vi "write_FP_data_to_fpga.vi"(8 "error in":errorcluster, 10 "all rows":dbl[](array[numeric]), 11 "FPGA Interface":T1) -> (0 "error out":errorcluster, 3 "elements left":i32=1)   [LabVIEW 2017]
uses:
  fpga_interface_types/HOST_to_FPGA_fp_FIFO_interface.ctl
  <vilib>/Utility/error.llb/Error Cluster From Error Code.vi
  <vilib>/rvi/errors/niLvFpgaAdjustHostInterfaceError.vi
  <vilib>/rvi/interface/nirviMethod/nirviMethod.xnode
  <vilib>/FPGAPlugInAG/Dynamic/niLvFpga_WriteFifo_Dynamic.vi
  <vilib>/rvi/errors/niLvFpgaMergeErrorWithErrorCode.vi
panel:
  out "Numeric":i32
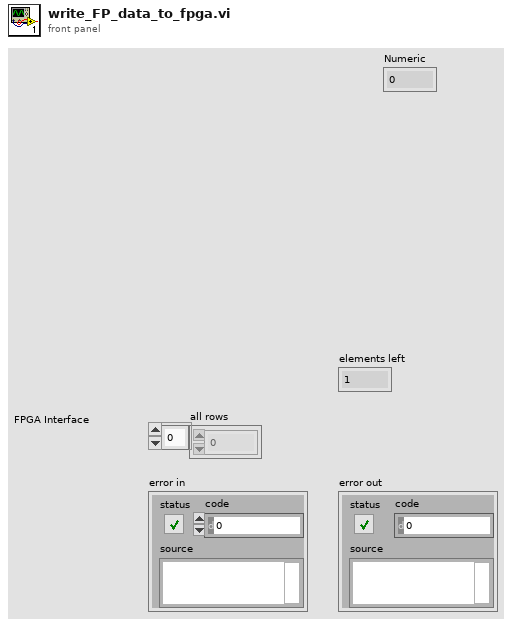
[diagram p1: front panel]
types:
  T1 = typedef "HOST_to_FPGA_fp_FIFO_interface.ctl" = refnum<k20>
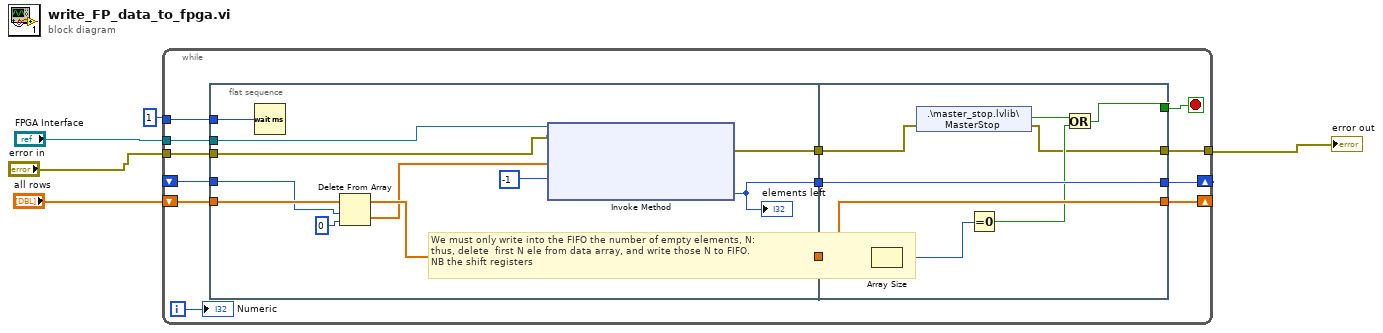
[diagram p0: block diagram]
diagram:
  n1 = while {
    tunnel: [w16] -> w4
    tunnel: 1 -> [w18]
    shift-right: [w11] -> _
    shift-left: _ -> [w15]
    shift-right: [w9] -> _
    shift-left: "all rows" -> [w17]
    tunnel: "FPGA Interface" -> [w8]
    tunnel: "error in" -> [w7]
    i -> [w6]
    stop <- w12 stop-if-true
    n2 = flat-sequence {
      tunnel: w18 -> [w29]
      tunnel: w17 -> [w26]
      tunnel: w15 -> [w25]
      tunnel: [w23] -> w14
      tunnel: [w20] -> w13
      tunnel: [w27] -> w10
      tunnel: w8 -> [w24]
      tunnel: w7 -> [w22]
      tunnel: [w37] -> w11
      tunnel: [w30] -> w16
      tunnel: w14 -> [w31]
      tunnel: w13 -> [w37]
      tunnel: [w33] -> w12
      tunnel: w10 -> [w35]
      tunnel: [w35] -> w9
      frame #0 {
        # "We must only write into the FIFO the number of empty elements, N:\nthus, delete  first N ele from data array, and write those N to FIFO.\nNB the shift registers"
        n3 = Wait (ms)(milliseconds to wait=w29) -> ()  [unwired: 1 out]
        n4 = Delete From Array(array=w26, length=w25, index=0) -> (deleted portion=w19:dbl[], array with subset deleted=w27:dbl[])
        n5 = xnode "Invoke Method"("FPGA VI Reference In"=w24, "error in"=w22, "Data"=w19, "Timeout (ms)"=-1) -> ("error out"=w23:errorcluster, "Empty Elements Remaining"=w20:u32)  [unwired: 1 out]
        "elements left" <- w20
      }
      frame #1 {
        n6 = Array Size(array=w35) -> (size(s)=w36:i32)
        n7 = shared-variable ".\\master_stop.lvlib\\MasterStop"(error in=w31) -> (w32:bool, error out=w30:errorcluster)
        n8 = Equal To 0?(x=w36) -> (x = 0?=w34:bool)
        n9 = Or(x=w32, y=w34) -> (x .or. y?=w33:bool)
      }
    }
    "Numeric" <- w6
  }
  "error out" <- w4
